vi "Lab 2 Zeke Carrasco.vi"() -> ()   [LabVIEW 2010]
uses:
  <vilib>/Utility/file.llb/Write To Spreadsheet File (DBL).vi
  <vilib>/Analysis/NI_AALBase.lvlib
panel:
  in  "Save File (up is \"yes\")?":bool
  in  "file path (dialog if empty)":path
  out "XY Graph":T1(graph)
  in  "Histrogram Invervals":i32
  out "1D Graph of Numbers with Exp. Dist.":dbl[](graph)
  in  "Expected Average Value":dbl
  in  "Number of Elements":i32
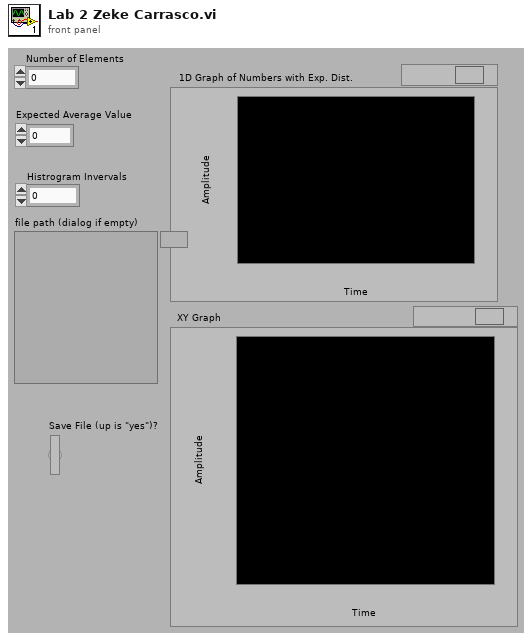
[diagram p1: front panel]
types:
  T1 = cluster{"X Values":dbl[], "Histogram: h(x)":i32[]}
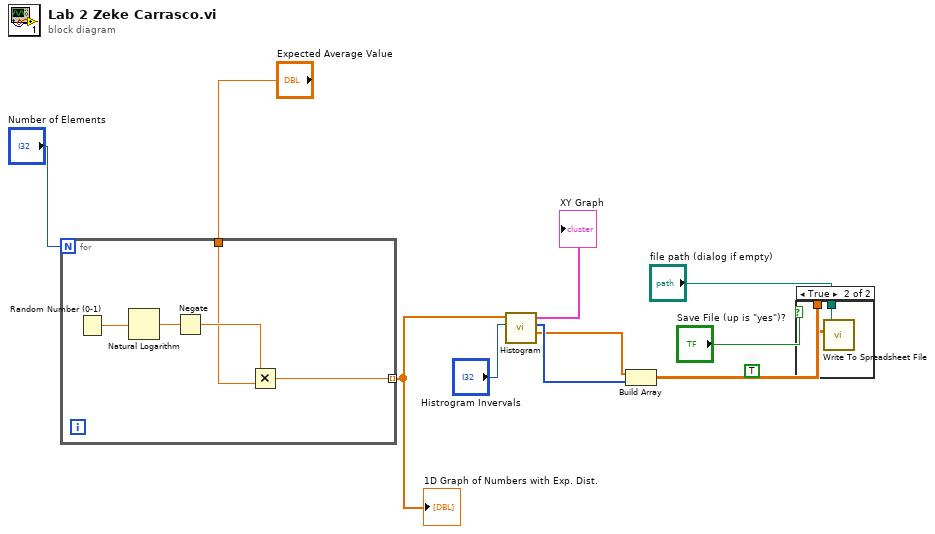
[diagram p0: block diagram]
diagram:
  (unwired) TRUE ("transpose? (no:F)")
  n1 = for {
    N: "Number of Elements" -> [_]
    tunnel: "Expected Average Value" -> [w12]
    tunnel: [w11] -> w7 mode=indexing
    n2 = Random Number (0-1)() -> (number: 0 to 1=w15:dbl)
    n3 = Natural Logarithm(1:w15) -> (0:w14:dbl)
    n4 = Negate(x=w14) -> (-x=w13:dbl)
    n5 = Multiply(x=w13, y=w12) -> (x*y=w11:dbl)
  }
  "1D Graph of Numbers with Exp. Dist." <- w7
  n6 = call <vilib>:"Histogram.vi"("intervals"="Histrogram Invervals", "X"=w7) -> ("X Values"=w4:dbl[], "Histogram: h(x)"=w5:i32[], "Histogram Graph"=→"XY Graph":T1)  [unwired: 6 in, 1 out]
  n7 = Build Array(w4, w5) -> (w2:dbl[][])
  n8 = case shown="True" "Save File (up is \"yes\")?" {
    tunnel: w2 -> [_ w17]
    tunnel: "file path (dialog if empty)" -> [_ w16]
    frame False {
    }
    frame True {
      n9 = call-poly <vilib>:"Write To Spreadsheet File.vi"("2D data"=w17, "file path (dialog if empty)"=w16) -> ()  [unwired: 6 in, 1 out]
    }
  }
